vi "4 roads.vi"() -> ()   [LabVIEW 2020]
panel:
  in  "Accident":bool
  out "Boolean 12":bool
  out "Boolean 11":bool
  out "Boolean 10":bool
  out "Boolean 9":bool
  out "Boolean 8":bool
  out "Boolean 7":bool
  out "Boolean 6":bool
  out "Boolean 5":bool
  out "Boolean 4":bool
  out "Boolean 3":bool
  out "Boolean 2":bool
  out "Boolean":bool
  in  "stop":bool
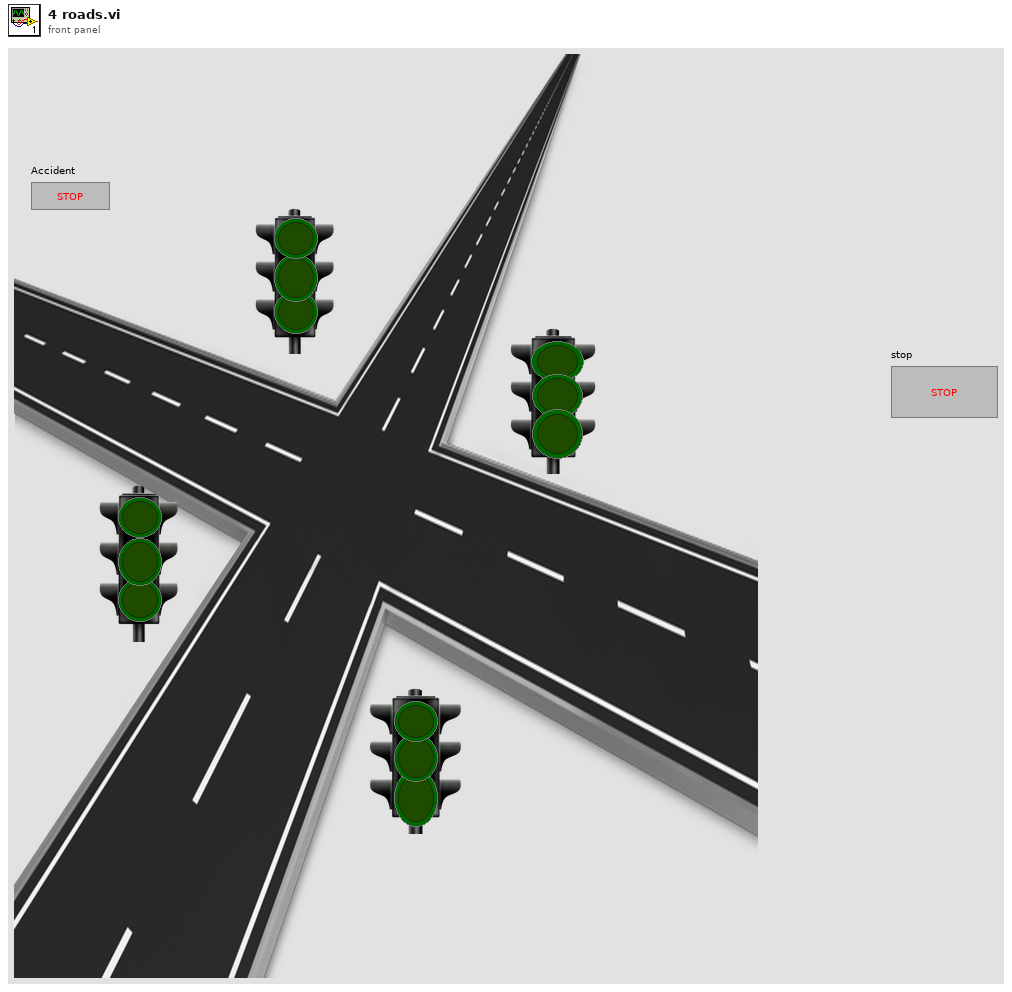
[diagram p1: front panel]
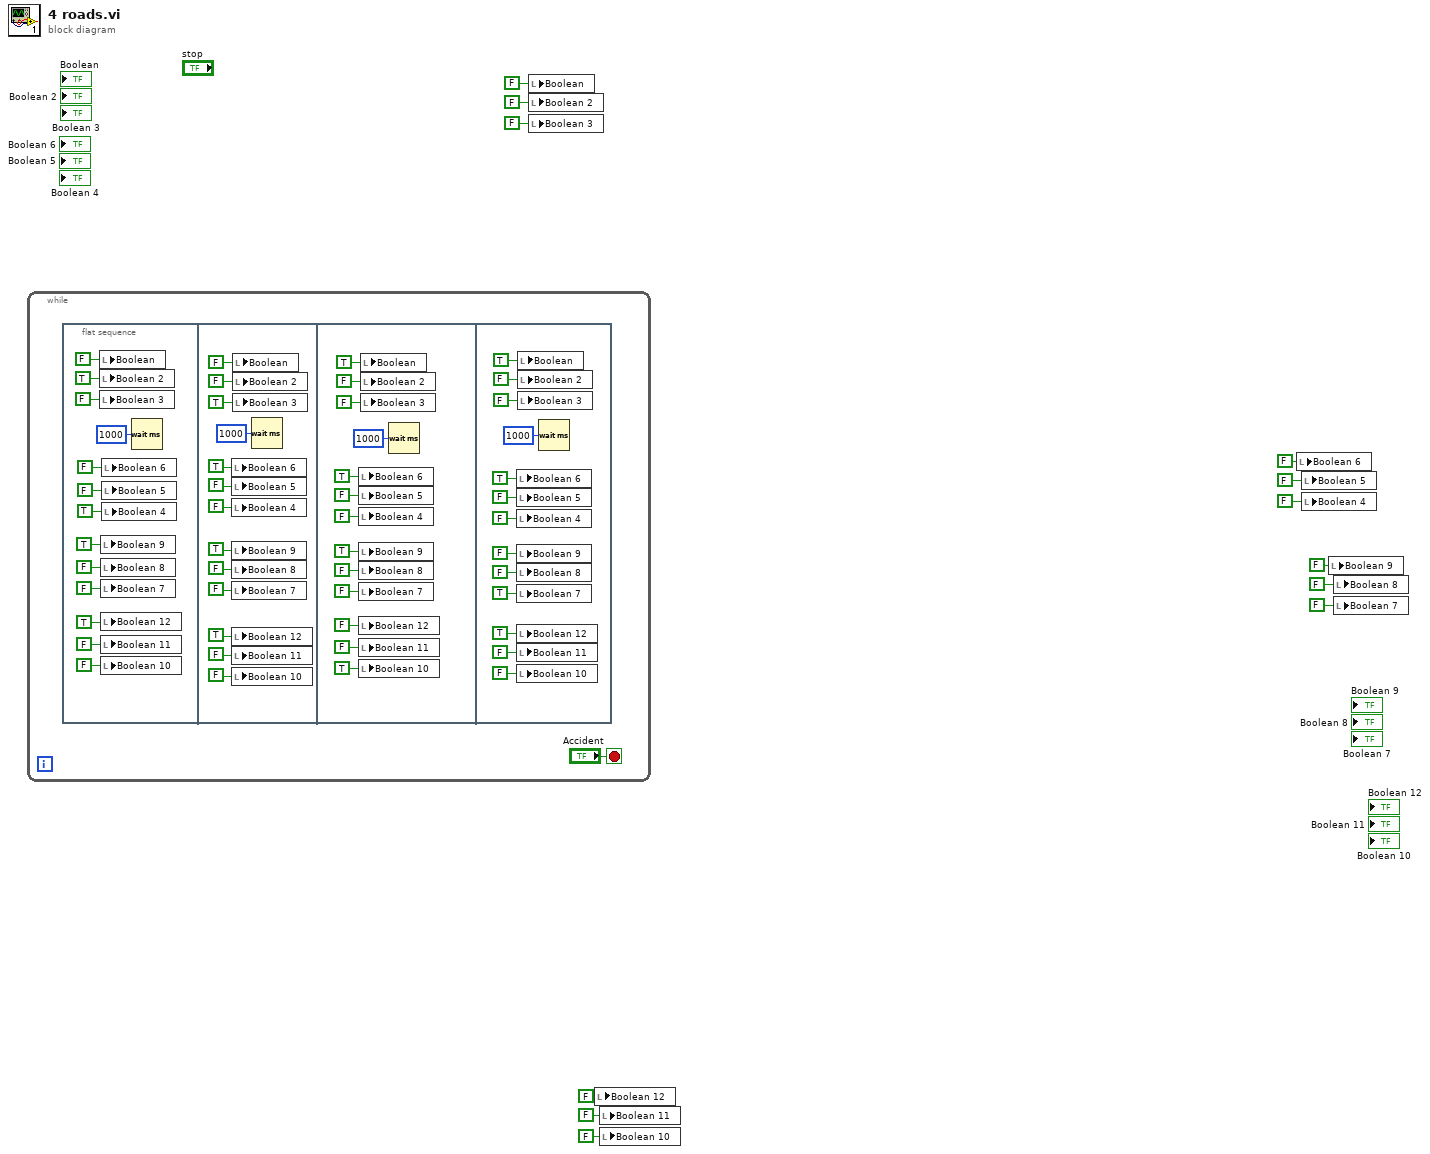
[diagram p0: block diagram]
diagram:
  n1 = while {
    stop <- "Accident" stop-if-true
    n2 = flat-sequence {
      frame #0 {
        n3 = local write "Boolean"(FALSE ("Boolean")) -> ()
        n4 = local write "Boolean 2"(TRUE ("Boolean 2")) -> ()
        n5 = local write "Boolean 3"(FALSE ("Boolean 3")) -> ()
        n6 = local write "Boolean 9"(TRUE ("Boolean")) -> ()
        n7 = local write "Boolean 8"(FALSE ("Boolean 2")) -> ()
        n8 = local write "Boolean 7"(FALSE ("Boolean 3")) -> ()
        n9 = local write "Boolean 12"(TRUE ("Boolean")) -> ()
        n10 = local write "Boolean 11"(FALSE ("Boolean 2")) -> ()
        n11 = local write "Boolean 10"(FALSE ("Boolean 3")) -> ()
        n12 = local write "Boolean 6"(FALSE ("Boolean")) -> ()
        n13 = local write "Boolean 5"(FALSE ("Boolean 2")) -> ()
        n14 = local write "Boolean 4"(TRUE ("Boolean 3")) -> ()
        n15 = Wait (ms)(milliseconds to wait=u32 1000 ("millisecond timer value")) -> ()  [unwired: 1 out]
      }
      frame #1 {
        n16 = local write "Boolean 6"(TRUE ("Boolean")) -> ()
        n17 = local write "Boolean 5"(FALSE ("Boolean 2")) -> ()
        n18 = local write "Boolean 4"(FALSE ("Boolean 3")) -> ()
        n19 = local write "Boolean 9"(TRUE ("Boolean")) -> ()
        n20 = local write "Boolean 8"(FALSE ("Boolean 2")) -> ()
        n21 = local write "Boolean 7"(FALSE ("Boolean 3")) -> ()
        n22 = local write "Boolean 12"(TRUE ("Boolean")) -> ()
        n23 = local write "Boolean 11"(FALSE ("Boolean 2")) -> ()
        n24 = local write "Boolean 10"(FALSE ("Boolean 3")) -> ()
        n25 = local write "Boolean"(FALSE ("Boolean")) -> ()
        n26 = local write "Boolean 2"(FALSE ("Boolean 2")) -> ()
        n27 = local write "Boolean 3"(TRUE ("Boolean 3")) -> ()
        n28 = Wait (ms)(milliseconds to wait=u32 1000 ("millisecond timer value")) -> ()  [unwired: 1 out]
      }
      frame #2 {
        n29 = local write "Boolean 6"(TRUE ("Boolean")) -> ()
        n30 = local write "Boolean 5"(FALSE ("Boolean 2")) -> ()
        n31 = local write "Boolean 4"(FALSE ("Boolean 3")) -> ()
        n32 = local write "Boolean 9"(TRUE ("Boolean")) -> ()
        n33 = local write "Boolean 8"(FALSE ("Boolean 2")) -> ()
        n34 = local write "Boolean 7"(FALSE ("Boolean 3")) -> ()
        n35 = local write "Boolean 12"(FALSE ("Boolean")) -> ()
        n36 = local write "Boolean 11"(FALSE ("Boolean 2")) -> ()
        n37 = local write "Boolean 10"(TRUE ("Boolean 3")) -> ()
        n38 = local write "Boolean"(TRUE ("Boolean")) -> ()
        n39 = local write "Boolean 2"(FALSE ("Boolean 2")) -> ()
        n40 = local write "Boolean 3"(FALSE ("Boolean 3")) -> ()
        n41 = Wait (ms)(milliseconds to wait=u32 1000 ("millisecond timer value")) -> ()  [unwired: 1 out]
      }
      frame #3 {
        n42 = local write "Boolean 6"(TRUE ("Boolean")) -> ()
        n43 = local write "Boolean 5"(FALSE ("Boolean 2")) -> ()
        n44 = local write "Boolean 4"(FALSE ("Boolean 3")) -> ()
        n45 = local write "Boolean 9"(FALSE ("Boolean")) -> ()
        n46 = local write "Boolean 8"(FALSE ("Boolean 2")) -> ()
        n47 = local write "Boolean 7"(TRUE ("Boolean 3")) -> ()
        n48 = local write "Boolean 12"(TRUE ("Boolean")) -> ()
        n49 = local write "Boolean 11"(FALSE ("Boolean 2")) -> ()
        n50 = local write "Boolean 10"(FALSE ("Boolean 3")) -> ()
        n51 = local write "Boolean"(TRUE ("Boolean")) -> ()
        n52 = local write "Boolean 2"(FALSE ("Boolean 2")) -> ()
        n53 = local write "Boolean 3"(FALSE ("Boolean 3")) -> ()
        n54 = Wait (ms)(milliseconds to wait=u32 1000 ("millisecond timer value")) -> ()  [unwired: 1 out]
      }
    }
  }
  n55 = local write "Boolean"(FALSE ("Boolean")) -> ()
  n56 = local write "Boolean 2"(FALSE ("Boolean 2")) -> ()
  n57 = local write "Boolean 3"(FALSE ("Boolean 3")) -> ()
  n58 = local write "Boolean 12"(FALSE ("Boolean")) -> ()
  n59 = local write "Boolean 11"(FALSE ("Boolean 2")) -> ()
  n60 = local write "Boolean 10"(FALSE ("Boolean 3")) -> ()
  n61 = local write "Boolean 6"(FALSE ("Boolean")) -> ()
  n62 = local write "Boolean 5"(FALSE ("Boolean 2")) -> ()
  n63 = local write "Boolean 4"(FALSE ("Boolean 3")) -> ()
  n64 = local write "Boolean 9"(FALSE ("Boolean")) -> ()
  n65 = local write "Boolean 8"(FALSE ("Boolean 2")) -> ()
  n66 = local write "Boolean 7"(FALSE ("Boolean 3")) -> ()
